vi "Write INI File Path.vi"(8 "error in (no error)":errorcluster, 10 "INI File Path":path, 11 "Control Info in":refnum<class "Control Info.lvclass">) -> (0 "error out":errorcluster, 3 "Control Info out":refnum<class "Control Info.lvclass">)   [LabVIEW 2017, in "Localization.lvlib" / "Control Info.lvclass"]
doc: "Write the INI file path to the class data.\n\nChoose Movement Consulting, LLC"
uses:
  Control Info.lvclass
  Control Info.lvclass/Control Info.ctl
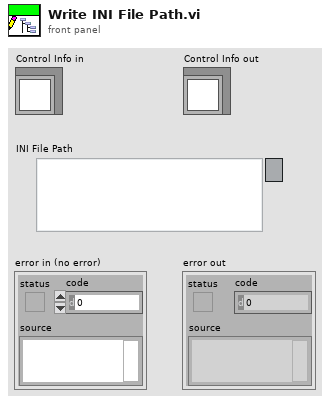
[diagram p1: front panel]
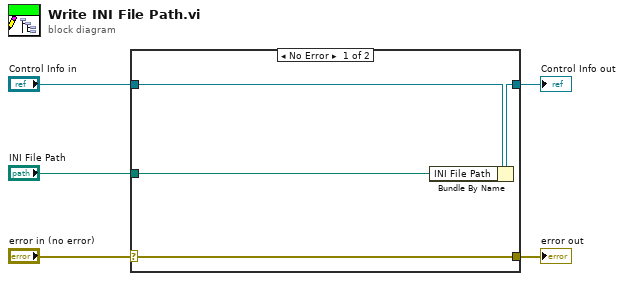
[diagram p0: block diagram]
diagram:
  n1 = case shown="No Error" "error in (no error)" {
    selector: "error in (no error)" -> [w9 w10]
    tunnel: [w9 w10] -> w4
    tunnel: [w7 w11] -> w2
    tunnel: "Control Info in" -> [w8 w11]
    tunnel: "INI File Path" -> [w6 _]
    frame No Error {
      n2 = Bundle By Name(cluster=w8, "INI File Path"=w6) -> (w7:refnum<class "Control Info.lvclass">)
    }
    frame Error {
    }
  }
  "error out" <- w4
  "Control Info out" <- w2
